vi "close.vi"(8 "error in (no error)":errorcluster, 11 "3_amp_volt in":refnum<class "3_amp_volt.lvclass">) -> (0 "error out":errorcluster, 3 "3_amp_volt out":refnum<class "3_amp_volt.lvclass">)   [LabVIEW 2018, in "3_amp_volt.lvclass"]
uses:
  3_amp_volt.lvclass
  3_amp_volt.lvclass/3_amp_volt.ctl
  <vilib>/Plasmionique/MB Master/MB_Master_Serial/MB_Master_Serial.lvclass
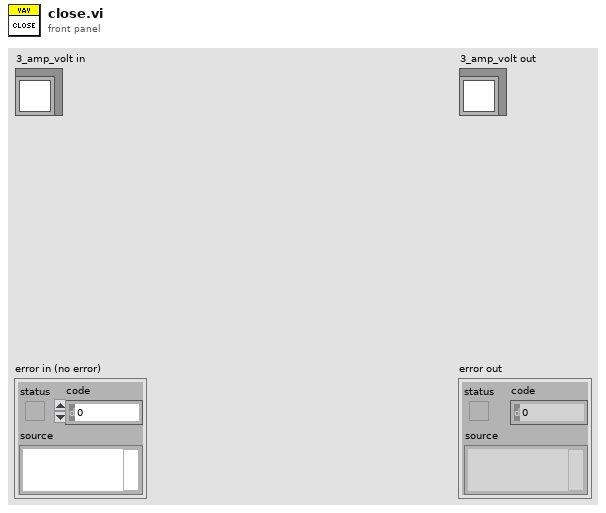
[diagram p1: front panel]
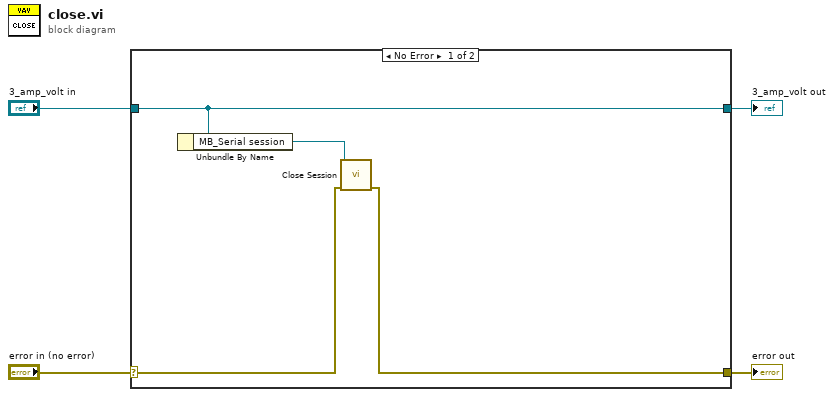
[diagram p0: block diagram]
diagram:
  n1 = case shown="No Error" "error in (no error)" {
    selector: "error in (no error)" -> [w6 w10]
    tunnel: [w5 w10] -> w3
    tunnel: [w8 w9] -> w1
    tunnel: "3_amp_volt in" -> [w8 w9]
    frame No Error {
      n2 = Unbundle By Name(w8) -> ("MB_Serial session"=w7:refnum<class "MB_Master_Serial.lvclass">)
      n3 = call-dynamic "Close Session.vi"("error in (no error)"=w6, "MB_Serial session"=w7) -> ("error out"=w5:errorcluster)  [unwired: 9 in]
    }
    frame Error {
    }
  }
  "error out" <- w3
  "3_amp_volt out" <- w1
